vi "Handle Error.vi"(8 "error in (no error)":errorcluster, 11 "Command in":refnum<class "Command.lvclass">) -> (0 "error out":errorcluster, 2 "stop actor?":bool=TRUE, 3 "Command out":refnum<class "Command.lvclass">)   [LabVIEW 2013, in "Robot Actors.lvlib" / "Command.lvlib" / "Command.lvclass"]
doc: "(<B>Filename</B>: Actor Framework.lvlib:Actor.lvclass:Handle Error.vi)\n\nDefines how the actor handles an error that occurred while processing a message.\n\nBy default, this method does nothing except stop the actor. This method also treats error code 43 (coming from <B>error in</B>) as a sign that the actor shut down normally. In this situation, the Handle Error method does not return the error on <B>error out</B>, meaning the actor's caller will not receive it. All other error codes will be returned on <B>error out</B>.\n\nA descendant class may override this method to change this behavior."
uses:
  Command.lvclass
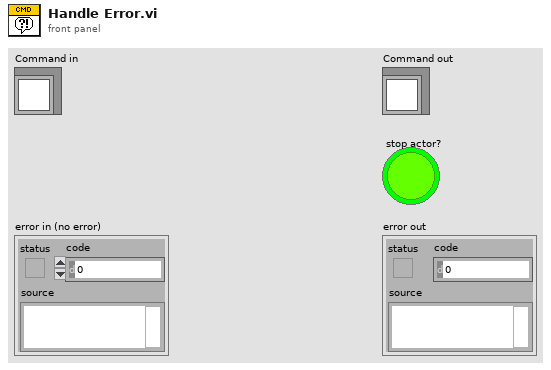
[diagram p1: front panel]
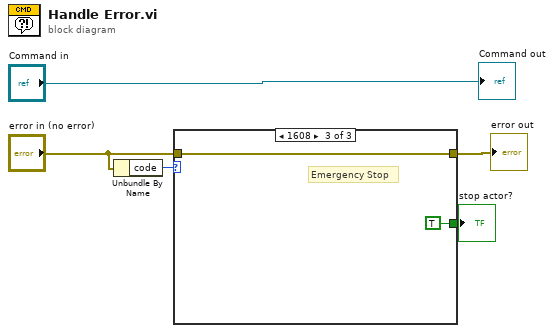
[diagram p0: block diagram]
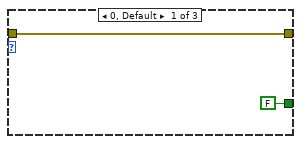
[diagram p2: hidden frame]
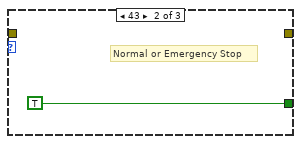
[diagram p3: hidden frame]
diagram:
  n1 = Unbundle By Name("error in (no error)") -> ("code"=w5:i32)
  n2 = case shown="1608" w5 {
    tunnel: [FALSE ("stop actor?") TRUE ("stop actor?") TRUE ("stop actor?")] -> w4
    tunnel: "error in (no error)" -> [w6 _ w9]
    tunnel: [w6 _ w9] -> w2
    frame 0, Default {
    }
    frame 43 {
      # "Normal or Emergency Stop"
    }
    frame 1608 {
      # "Emergency Stop"
    }
  }
  "error out" <- w2
  "stop actor?" <- w4
  "Command out" <- "Command in"
